vi "Agilent VNA Read Learn String.vi"(7 "Agilent VNA":T1={"Model"="8510", "Serial"="", "Firmware"="", "Learn String"=""}, 8 "error in (no error)":errorcluster, 11 "VISA Resource Name":refnum<visa-resource-name>="GPIB0::16::INSTR") -> (0 "error out":errorcluster, 2 "Learn String":string, 3 "dup VISA Resource Name":refnum<visa-resource-name>="GPIB0::16::INSTR")   [LabVIEW 2011]
uses:
  TypeDefs/Agilent VNA Instrument Info.ctl
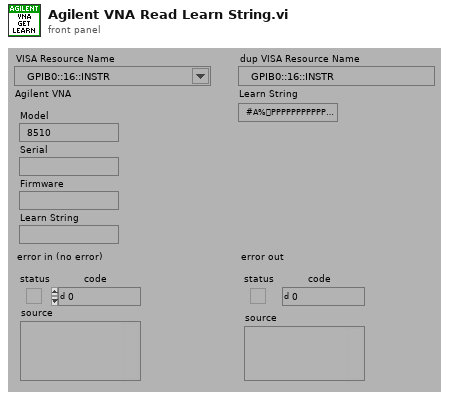
[diagram p1: front panel]
types:
  T1 = typedef "Agilent VNA Instrument Info.ctl" = cluster{"Model":string, "Serial":string, "Firmware":string, "Learn String":string}
  T2 = typedef "Agilent VNA Model.ctl" = enum16{"Not Supported", "8510X", "8719X", "8720X", "8722X", "8753X", "ENA", "PNA", "Field Fox"}
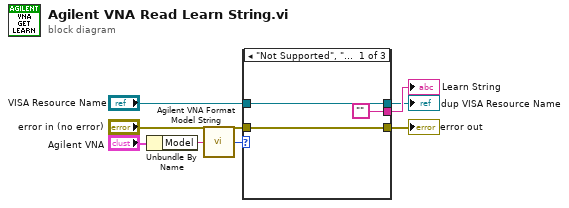
[diagram p0: block diagram]
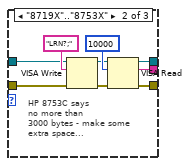
[diagram p2: hidden frame]
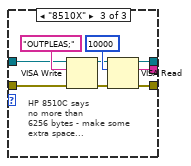
[diagram p3: hidden frame]
diagram:
  n1 = Unbundle By Name("Agilent VNA") -> ("Model"=w1:string)
  n2 = call "Agilent VNA Format Model String.vi"("Model"=w1) -> ("Model"=w3:T2)
  n3 = case shown="\"Not Supported\", \"ENA\"..\"Field Fox\"" w3 {
    tunnel: "VISA Resource Name" -> [w11 w16 w25]
    tunnel: ["" w15 w24] -> w7
    tunnel: "error in (no error)" -> [w10 w14 w23]
    tunnel: [w10 w13 w22] -> w5
    tunnel: [w11 w12 w21] -> w4
    frame "Not Supported", "ENA".."Field Fox" {
    }
    frame "8719X".."8753X" {
      # "HP 8753C says\nno more than\n3000 bytes - make some\nextra space..."
      n4 = VISA Write(VISA resource name=w16, write buffer="LRN?;", error in (no error)=w14) -> (VISA resource name out=w17:refnum<visa-resource-name>, error out=w19:errorcluster)  [unwired: 1 out]
      n5 = VISA Read(VISA resource name=w17, byte count=u32 10000, error in (no error)=w19) -> (VISA resource name out=w12:refnum<visa-resource-name>, read buffer=w15:string, error out=w13:errorcluster)  [unwired: 1 out]
    }
    frame "8510X" {
      # "HP 8510C says\nno more than\n6256 bytes - make some\nextra space..."
      n6 = VISA Write(VISA resource name=w25, write buffer="OUTPLEAS;", error in (no error)=w23) -> (VISA resource name out=w26:refnum<visa-resource-name>, error out=w28:errorcluster)  [unwired: 1 out]
      n7 = VISA Read(VISA resource name=w26, byte count=u32 10000, error in (no error)=w28) -> (VISA resource name out=w21:refnum<visa-resource-name>, read buffer=w24:string, error out=w22:errorcluster)  [unwired: 1 out]
    }
  }
  "error out" <- w5
  "dup VISA Resource Name" <- w4
  "Learn String" <- w7
